vi "ActionVIOnDownload.vi"(5 "System Definition Dir":path, 6 "IP address":string, 7 "Details Ref":refnum<vi>, 8 "error in (no error)":errorcluster, 10 "ftp session":T2, 11 "Device Item Ref in":T1 format="%.0x") -> (0 "error out":errorcluster, 2 "ftp session out":T2, 3 "Device Item Ref out":T1 format="%.0x")   [LabVIEW 2013, in "Diagnostics Addon System Explorer.lvlib"]
uses:
  Diagnostics Addon System Explorer.lvlib
  <vilib>/FTP/ftp0.llb/FTP Session.ctl
  <vilib>/NI Veristand/Custom Device API/Custom Device Item Ref.ctl
  Shared/GUID Lookup.vi
  Shared/Diagnostics Addon Shared.lvlib
  <vilib>/FTP/NI_FTP.lvlib
  <vilib>/NI Veristand/Custom Device API/Custom Device API.lvlib
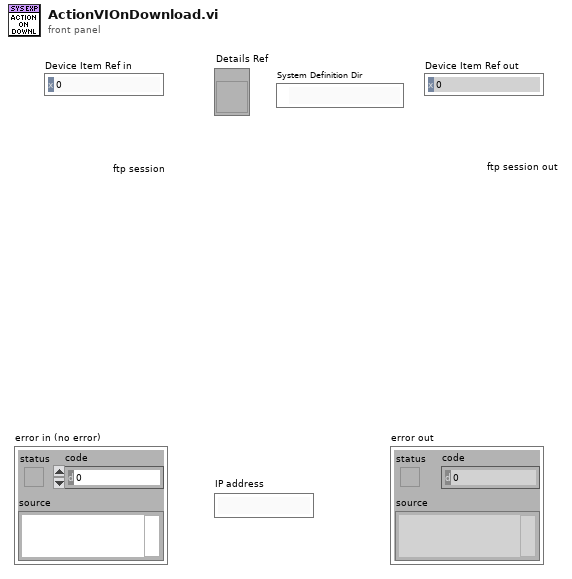
[diagram p1: front panel]
types:
  T1 = typedef "Custom Device API.lvlib/Custom Device Item Ref.ctl" = u64
  T2 = typedef "NI_FTP.lvlib/FTP Session.ctl" = refnum<k5>
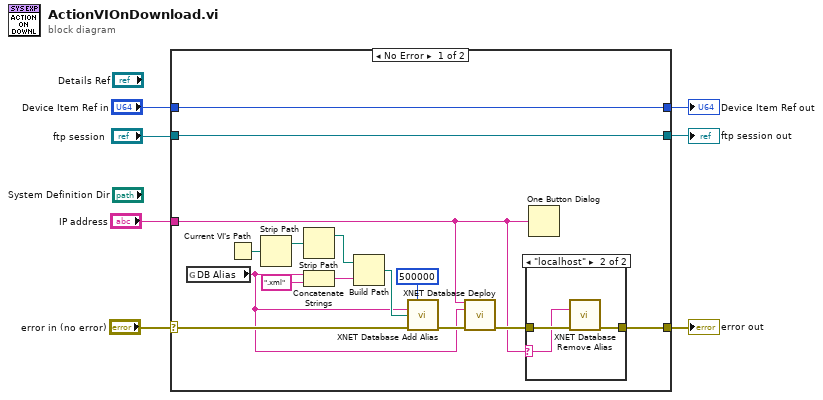
[diagram p0: block diagram]
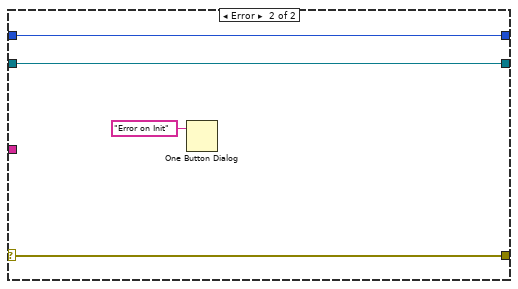
[diagram p3: hidden frame]
diagram:
  n1 = case shown="No Error" "error in (no error)" {
    selector: "error in (no error)" -> [w20 w30]
    tunnel: [w12 w30] -> w1
    tunnel: "ftp session" -> [w22 w29]
    tunnel: [w22 w29] -> w6
    tunnel: "Device Item Ref in" -> [w21 w28]
    tunnel: [w21 w28] -> w4
    tunnel: "IP address" -> [w8 _]
    frame No Error {
      n2 = global read "GUID Lookup.vi" "DB Alias"() -> (w9:string)
      n3 = Current VI's Path() -> (path=w19:path)
      n4 = Strip Path(path=w19) -> (stripped path=w15:path)  [unwired: 1 out]
      n5 = Strip Path(path=w15) -> (stripped path=w14:path)  [unwired: 1 out]
      n6 = Concatenate Strings(w9, ".xml" ("string")) -> (w17:string)
      n7 = Build Path(base path=w14, name or relative path=w17) -> (appended path=w13:path)
      n8 = call <vilib>:"XNET Database Add Alias.vi"("default baud rate (0)"=u32 500000, "alias"=w9, "filepath"=w13, "error in (no error)"=w20) -> ("error out"=w11:errorcluster)  [unwired: 11 in]
      n9 = call <vilib>:"XNET Database Deploy.vi"("IP address"=w8, "alias"=w9, "error in (no error)"=w11) -> ("error out"=w10:errorcluster)  [unwired: 11 in, 1 out]
      n10 = case shown="\"localhost\"" w8 {
        selector: w8 -> [_ w24]
        tunnel: [w23 w26] -> w12
        tunnel: w10 -> [w23 w25]
        frame "False", Default {
        }
        frame "localhost" {
          n11 = call <vilib>:"XNET Database Remove Alias.vi"("alias"=w24, "error in (no error)"=w25) -> ("error out"=w26:errorcluster)  [unwired: 13 in]
        }
      }
      n12 = One Button Dialog(message=w8) -> ()  [unwired: 1 in, 1 out]
    }
    frame Error {
      n13 = One Button Dialog(message="Error on Init") -> ()  [unwired: 1 in, 1 out]
    }
  }
  "error out" <- w1
  "ftp session out" <- w6
  "Device Item Ref out" <- w4
